vi "1.vi"() -> ()   [LabVIEW 2018]
panel:
  in  "stop":bool
  out "resultado":dbl
  in  "entrada 2":dbl(knob) scale=0.0..10.0
  in  "entrada 1":dbl(knob) scale=0.0..10.0
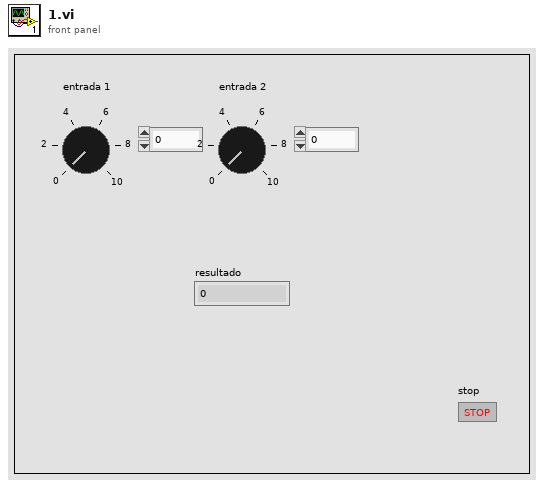
[diagram p1: front panel]
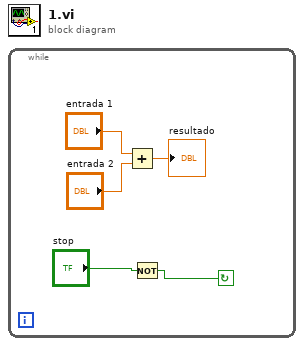
[diagram p0: block diagram]
diagram:
  n1 = while {
    stop <- w2 continue-if-true
    n2 = Add(x="entrada 1", y="entrada 2") -> (x+y=→"resultado":dbl)
    n3 = Not(x="stop") -> (.not. x?=w2:bool)
  }
